vi "sabertooth packetized set settings.vi"(1 "Data":u32, 2 "Command List":T1=15 items=["Min voltage"=2, "Max voltage"=3, "Serial Timeout"=14, "Baud Rate"=15, "Ramping"=16, "Deadband"=17], 3 "Sabertooth Addresses":T2=128 items=["Sabertooth 1"=128, "Sabertooth 2"=129, "Sabertooth 3"=130, "Sabertooth 4"=131, "Sabertooth 5"=132, "Sabertooth 6"=133, "Sabertooth 7"=134, "Sabertooth 8"=135]) -> (0 "msg out":string)   [LabVIEW 2018]
uses:
  controls/Sabertooth Address Select.ctl
  controls/Sabertooth Command Select.ctl
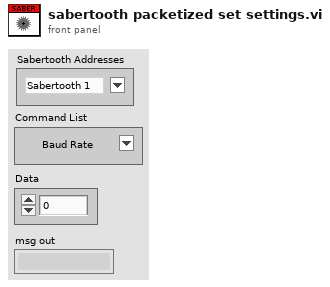
[diagram p1: front panel]
types:
  T1 = typedef "Sabertooth Command Select.ctl" = u8
  T2 = typedef "Sabertooth Address Select.ctl" = u8
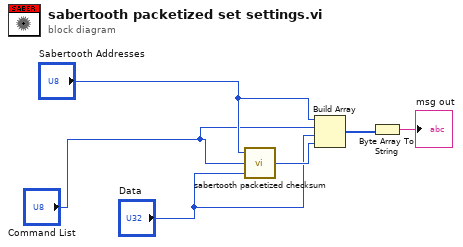
[diagram p0: block diagram]
diagram:
  n1 = call "sabertooth packetized checksum.vi"("Data"="Data", "Command"="Command List", "Address"="Sabertooth Addresses") -> ("Checksum"=w6:u8)
  n2 = Build Array("Sabertooth Addresses", "Command List", "Data", w6) -> (w3:u32[])
  n3 = Byte Array To String(unsigned byte array=w3) -> (string=→"msg out":string)
